vi "Analyze Data.vi"(8 "error in":errorcluster, 11 "ePAS in":refnum<class "ePAS.lvclass">) -> (0 "error out":errorcluster, 3 "ePAS out":refnum<class "ePAS.lvclass">)   [LabVIEW 2014, in "ePAS Library.lvlib" / "ePAS.lvclass"]
doc: "This is the core routine for PAS microphone data analysis. Here, the microphone data is retrieved from each of the cells. In both cases, the time domain signal will be transformed to the frequency domain. If the speaker is on (<B>Spk Pos</B> == TRUE), then the frequency domain signal will be squared to obtain the power and a Lorentzian will be fit to the data to retrieve the resonant characteristics of the cell. If the speaker is off (<B>Spk Pos</B> == FALSE), then the amplitude will be used to calculate the integrated area of the signal. In every case, the implementation has the ability to decimate the data for transmission of the waveforms over a network line."
uses:
  ePAS.lvclass
  reusable/Instrument/Instrument.lvclass/Instrument.ctl
  reusable/PAS/Data/Main/PAS Data.lvclass
  Commands/Change PAS Laser Frequency/Change Laser Frequency.lvclass
  Commands/Change PAS Laser Frequency/Change Laser Frequency.lvclass/Change Laser Frequency.ctl
  reusable/Instrument/Read CMD.vi
  Commands/Change PAS Laser Frequency/Write f0.vi
  reusable/Instrument/Read ExtCom.vi
  reusable/Instrument/Read Data.vi
  reusable/PAS/Main/Get Speaker State.vi
  reusable/PAS/Data/Main/Read CellData.vi
  reusable/PAS/Data/Cell/Read f0.vi
  reusable/Data/Data.lvclass
  reusable/PAS/Data/Cell/PAS Cell Data.lvclass
  reusable/Command/Command.lvclass
  reusable/PAS/Main/PAS.lvclass
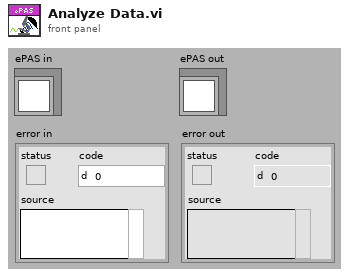
[diagram p1: front panel]
types:
  T1 = cluster{"tag":string, "section":string, "data":variant}
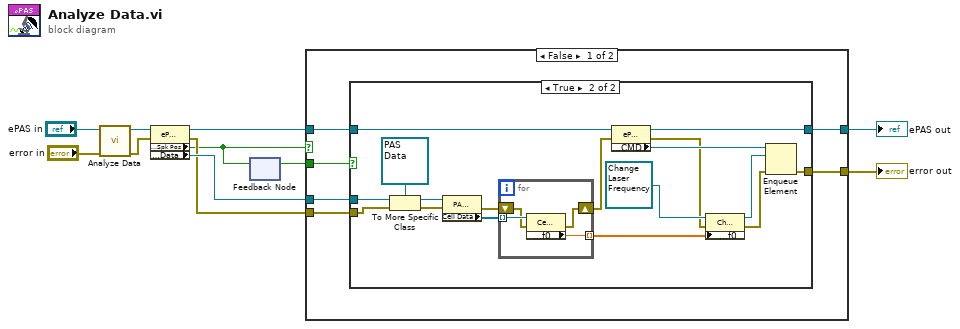
[diagram p0: block diagram]
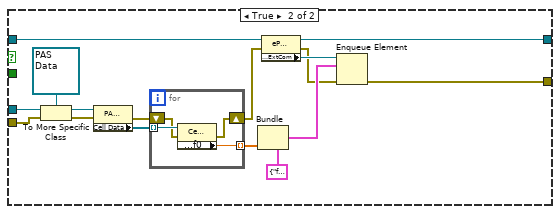
[diagram p3: hidden frame]
diagram:
  n1 = call-parent "Analyze Data.vi"("error in"="error in", "PAS in"="ePAS in") -> ("error out"=w7:errorcluster, "PAS out"=w9:refnum<class "ePAS.lvclass">)  [unwired: 8 in]
  n2 = property class="ePAS"(reference=w9, error in=w7) -> (reference out=w2:refnum<class "ePAS.lvclass">, error out=w6:errorcluster, "Data Access:Spk Pos"=w4:bool, "Accessors:Data"=w8:refnum<class "Data.lvclass">)
  n3 = feedback-in #1(w4) -> ()
  n4 = feedback #1() -> (w3:bool)  [unwired: 1 in]
  n5 = case shown="False" w4 {
    tunnel: w8 -> [w16 w53]
    tunnel: w6 -> [w15 w48]
    tunnel: [w14 w46] -> w5
    tunnel: w3 -> [w17 _]
    tunnel: w2 -> [w13 w45]
    tunnel: [w12 w43] -> w1
    frame False {
      n6 = case shown="True" w17 {
        tunnel: w16 -> [_ w31]
        tunnel: w15 -> [w19 w30]
        tunnel: [w19 w21] -> w14
        tunnel: w13 -> [w18 w29]
        tunnel: [w18 w20] -> w12
        frame False {
        }
        frame True {
          n7 = To More Specific Class(target class=refnum<class "PAS Data.lvclass"> refnum ("PAS Library.lvlib:PAS Data"), reference=w31, error in=w30) -> (specific class reference=w34:refnum<class "PAS Data.lvclass">, error out=w36:errorcluster)
          n8 = property class="PAS Data"(reference=w34, error in=w36) -> (error out=w32:errorcluster, "Cell Data"=w33:refnum<class "PAS Cell Data.lvclass">[])  [unwired: 1 out]
          n9 = for {
            tunnel: w33 -> [w40] mode=indexing
            tunnel: [w39] -> w25 mode=indexing
            shift-right: [w37] -> w28
            shift-left: w32 -> [w38]
            n10 = property class="Cell Data"(reference=w40, error in=w38) -> (error out=w37:errorcluster, "Accessors:f0"=w39:sgl)  [unwired: 1 out]
          }
          n11 = property class="ePAS"(reference=w29, error in=w28) -> (reference out=w20:refnum<class "ePAS.lvclass">, error out=w23:errorcluster, "Accessors:CMD"=w27:refnum<queue>)
          n12 = property class="Change Laser Frequency.lvclass"(reference=refnum<class "Change Laser Frequency.lvclass"> refnum ("ePAS Library.lvlib:Change Laser Frequency.lvclass"), error in=w23, "Accessors:f0"=w25) -> (reference out=w24:refnum<class "Change Laser Frequency.lvclass">, error out=w22:errorcluster)
          n13 = Enqueue Element(queue=w27, element=w24, error in (no error)=w22) -> (error out=w21:errorcluster)  [unwired: 1 in, 2 out]
        }
      }
    }
    frame True {
      n14 = To More Specific Class(target class=refnum<class "PAS Data.lvclass"> refnum ("PAS Library.lvlib:PAS Data"), reference=w53, error in=w48) -> (specific class reference=w51:refnum<class "PAS Data.lvclass">, error out=w54:errorcluster)
      n15 = property class="PAS Data"(reference=w51, error in=w54) -> (error out=w47:errorcluster, "Cell Data"=w50:refnum<class "PAS Cell Data.lvclass">[])  [unwired: 1 out]
      n16 = for {
        tunnel: w50 -> [w60] mode=indexing
        tunnel: [w59] -> w49 mode=indexing
        shift-right: [w57] -> w42
        shift-left: w47 -> [w58]
        n17 = property class="Cell Data"(reference=w60, error in=w58) -> (error out=w57:errorcluster, "Accessors:f0"=w59:sgl)  [unwired: 1 out]
      }
      n18 = Bundle(cluster=T1 {"tag"="f0", "section"="pas.las", "data"=variant} ("element"), "data"=w49) -> (w55:T1)  [unwired: 2 in]
      n19 = property class="ePAS"(reference=w45, error in=w42) -> (reference out=w43:refnum<class "ePAS.lvclass">, error out=w41:errorcluster, "Accessors:ExtCom"=w44:refnum<queue>)
      n20 = Enqueue Element(queue=w44, element=w55, error in (no error)=w41) -> (error out=w46:errorcluster)  [unwired: 1 in, 2 out]
    }
  }
  "error out" <- w5
  "ePAS out" <- w1
